vi "simulateRun.vi"() -> ()   [LabVIEW 2017]
uses:
  Settings/Settings-Control.ctl
  Globals/measurementGlobal.vi
  Settings/Traverse-Settings-Global.vi
panel:
  out "Total Traverse Time (hr)":dbl
  out "Total Traverse Time (min)":dbl
  out "Settings":T1
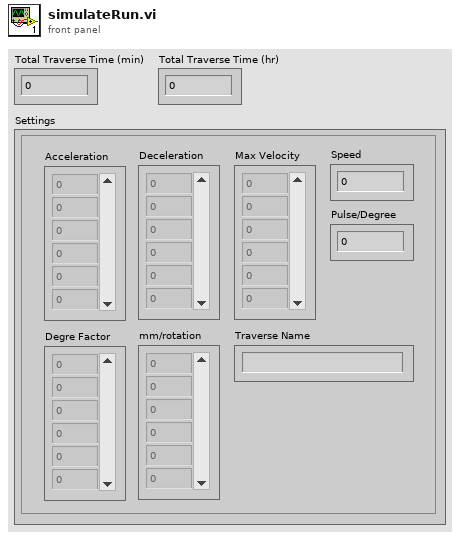
[diagram p1: front panel]
types:
  T1 = typedef "Settings-Control.ctl" = cluster{"Acceleration":dbl[], "Deceleration":dbl[], "Max Velocity":dbl[], "Speed":dbl, "Pulse/Degree":dbl, "Degre Factor":dbl[], "mm/rotation":dbl[], "Traverse Name":string}
  T2 = cluster{"TotalTime":dbl, "AccTime":dbl, "AccDist/Distance":dbl}[]
  T3 = cluster{"TotalTime":dbl, "AccTime":dbl, "AccDist/Distance":dbl}
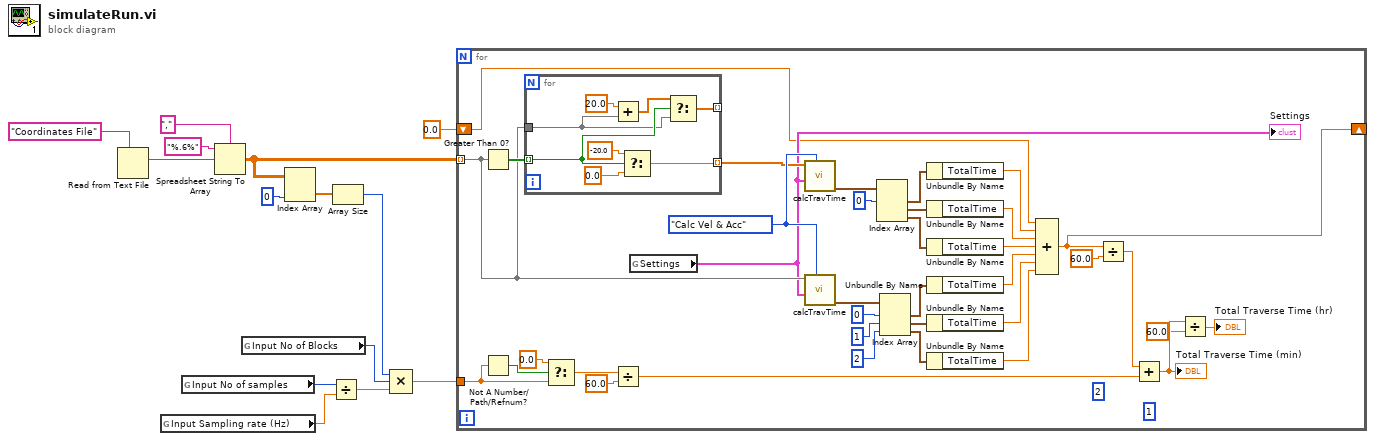
[diagram p0: block diagram]
diagram:
  n1 = Read from Text File(prompt (Open existing file)="Coordinates File") -> (text=w13:string)  [unwired: 3 in, 3 out]
  n2 = global read "measurementGlobal.vi" "Input Sampling rate (Hz)"() -> (w8:dbl)
  n3 = global read "measurementGlobal.vi" "Input No of samples"() -> (w9:i32)
  n4 = Spreadsheet String To Array(delimiter (Tab)=",", format string="%.6%", spreadsheet string=w13) -> (array=w3:dbl[][])  [unwired: 1 in]
  n5 = global read "measurementGlobal.vi" "Input No of Blocks"() -> (w7:i32)
  n6 = Index Array(array=w3, index (col)=0 ("disabled index (col)")) -> (element=w1:dbl[])  [unwired: 1 in]
  n7 = Divide(x=w9, y=w8) -> (x/y=w6:dbl)
  n8 = Array Size(array=w1) -> (size(s)=w5:i32)
  n9 = Compound Arithmetic op=MULTIPLY(w5, w7, w6) -> (w4:dbl)
  n10 = for {
    tunnel: w3 -> [w29] mode=indexing
    shift-right: [w26] -> _
    shift-left: 0.0 -> [w27]
    tunnel: w4 -> [w18]
    (unwired) 2 ("index")
    (unwired) 1 ("index")
    w49 = enum16{"Calc Vel & Acc", "Check Time"}."Calc Vel & Acc" ("Mode")
    n11 = Greater Than 0?(x=w29) -> (x > 0?=w50:bool[])
    n12 = Not A Number/Path/Refnum?(number/path/refnum=w18) -> (NaN/Path/Refnum?=w19:bool)
    n13 = for {
      tunnel: w50 -> [w53] mode=indexing
      tunnel: [w56] -> _ mode=indexing
      tunnel: [w52] -> w48 mode=indexing
      tunnel: w29 -> [w51]
      n14 = Add(x=20.0, y=w51) -> (x+y=w58:dbl[])
      n15 = Select(t=-20.0 ("x"), s=w53, f=0.0) -> (s? t:f=w52:dbl)
      n16 = Select(t=w58, s=w53, f=w51) -> (s? t:f=w56:dbl[])
    }
    n17 = Select(t=0.0, s=w19, f=w18) -> (s? t:f=w20:dbl)
    n18 = Divide(x=w20, y=60.0) -> (x/y=w22:dbl)
    n19 = global read "Traverse-Settings-Global.vi" "Settings"() -> (w28:T1)
    "Settings" <- w28
    n20 = call "calcTravTime.vi"("Mode"=w49, "Settings"=w28, "Total Distance"=w48) -> ("Channel Data"=w39:T2)  [unwired: 6 in, 2 out]
    n21 = call "calcTravTime.vi"("Mode"=w49, "Settings"=w28, "Total Distance"=w29) -> ("Channel Data"=w47:T2)  [unwired: 6 in, 2 out]
    n22 = Index Array(array=w39, index #1=0 ("index")) -> (element #1=w38:T3, element #2=w37:T3, element #3=w36:T3)  [unwired: 2 in]
    n23 = Index Array(array=w47, index #1=0 ("index"), index #2=1 ("index"), index #3=2 ("index")) -> (element #1=w43:T3, element #2=w42:T3, element #3=w41:T3)
    n24 = Unbundle By Name(w38) -> ("TotalTime"=w35:dbl)
    n25 = Unbundle By Name(w37) -> ("TotalTime"=w34:dbl)
    n26 = Unbundle By Name(w36) -> ("TotalTime"=w33:dbl)
    n27 = Unbundle By Name(w43) -> ("TotalTime"=w32:dbl)
    n28 = Unbundle By Name(w42) -> ("TotalTime"=w31:dbl)
    n29 = Unbundle By Name(w41) -> ("TotalTime"=w30:dbl)
    n30 = Compound Arithmetic op=ADD(w27, w35, w34, w33, w32, w31, w30) -> (w26:dbl)
    n31 = Divide(x=w26, y=60.0) -> (x/y=w23:dbl)
    n32 = Add(x=w23, y=w22) -> (x+y=w17:dbl)
    "Total Traverse Time (min)" <- w17
    n33 = Divide(x=w17, y=60.0) -> (x/y=→"Total Traverse Time (hr)":dbl)
  }
